vi "Create Gradient Color by Start and End Color DEMO.vi"() -> ()   [LabVIEW 2012, in "Picture Box Tools.lvlib"]
uses:
  Picture Box Tools.lvlib
panel:
  in  "End":u32(colorbox)
  in  "Start":u32(colorbox)=16448250
  out "1 Pix W - Color Box Array":u32[](array[colorbox])=[16448250, 16382457, 16316664, 16250871, 16185078, 16119285, 16053492, 15987699, 15921906, 15856113, 15790320, 15724527, 15658734, 15592941, 15527148, 15461355, 15395562, 15329769, 15263976, 15198183, 15132390, 15066597, 15000804, 14935011, 14869218, 14803425, 14803425, 14737632, 14671839, 14606046, 14540253, 14474460, 14408667, 14342874, 14277081, 14211288, 14145495, 14079702, 14013909, 13948116, 13882323, 13816530, 13750737, 13684944, 13619151, 13553358, 13487565, 13421772, 13355979, 13290186, 13224393, 13158600, 13092807, 13027014, 12961221, 12895428, 12829635, 12763842, 12698049, 12632256, 12566463, 12500670, 12434877, 12369084, 12303291, 12237498, 12171705, 12105912, 12040119, 11974326, 11908533, 11842740, 11776947, 11711154, 11645361, 11579568, 11513775, 11513775, 11447982, 11382189, 11316396, 11250603, 11184810, 11119017, 11053224, 10987431, 10921638, 10855845, 10790052, 10724259, 10658466, 10592673, 10526880, 10461087, 10395294, 10329501, 10263708, 10197915, 10132122, 10066329, 10000536, 9934743, 9868950, 9803157, 9737364, 9671571, 9605778, 9539985, 9474192, 9408399, 9342606, 9276813, 9211020, 9145227, 9079434, 9013641, 8947848, 8882055, 8816262, 8750469, 8684676, 8618883, 8553090, 8487297, 8421504, 8355711, 8289918, 8224125, 8224125, 8158332, 8092539, 8026746, 7960953, 7895160, 7829367, 7763574, 7697781, 7631988, 7566195, 7500402, 7434609, 7368816, 7303023, 7237230, 7171437, 7105644, 7039851, 6974058, 6908265, 6842472, 6776679, 6710886, 6645093, 6579300, 6513507, 6447714, 6381921, 6316128, 6250335, 6184542, 6118749, 6052956, 5987163, 5921370, 5855577, 5789784, 5723991, 5658198, 5592405, 5526612, 5460819, 5395026, 5329233, 5263440, 5197647, 5131854, 5066061, 5000268, 4934475, 4934475, 4868682, 4802889, 4737096, 4671303, 4605510, 4539717, 4473924, 4408131, 4342338, 4276545, 4210752, 4144959, 4079166, 4013373, 3947580, 3881787, 3815994, 3750201, 3684408, 3618615, 3552822, 3487029, 3421236, 3355443, 3289650, 3223857, 3158064, 3092271, 3026478, 2960685, 2894892, 2829099, 2763306, 2697513, 2631720, 2565927, 2500134, 2434341, 2368548, 2302755, 2236962, 2171169, 2105376, 2039583, 1973790, 1907997, 1842204, 1776411, 1710618, 1644825, 1644825, 1579032, 1513239, 1447446, 1381653, 1315860, 1250067, 1184274, 1118481, 1052688, 986895, 921102, 855309, 789516, 723723, 657930, 592137, 526344, 460551, 394758, 328965, 263172, 197379, 131586, 65793, 0]
  out "1 Pix H - Color Box Array":u32[](array[colorbox])=[16448250, 16382457, 16316664, 16250871, 16185078, 16119285, 16053492, 15987699, 15921906, 15856113, 15790320, 15724527, 15658734, 15592941, 15527148, 15461355, 15395562, 15329769, 15263976, 15198183, 15132390, 15066597, 15000804, 14935011, 14869218, 14803425, 14803425, 14737632, 14671839, 14606046, 14540253, 14474460, 14408667, 14342874, 14277081, 14211288, 14145495, 14079702, 14013909, 13948116, 13882323, 13816530, 13750737, 13684944, 13619151, 13553358, 13487565, 13421772, 13355979, 13290186, 13224393, 13158600, 13092807, 13027014, 12961221, 12895428, 12829635, 12763842, 12698049, 12632256, 12566463, 12500670, 12434877, 12369084, 12303291, 12237498, 12171705, 12105912, 12040119, 11974326, 11908533, 11842740, 11776947, 11711154, 11645361, 11579568, 11513775, 11513775, 11447982, 11382189, 11316396, 11250603, 11184810, 11119017, 11053224, 10987431, 10921638, 10855845, 10790052, 10724259, 10658466, 10592673, 10526880, 10461087, 10395294, 10329501, 10263708, 10197915, 10132122, 10066329, 10000536, 9934743, 9868950, 9803157, 9737364, 9671571, 9605778, 9539985, 9474192, 9408399, 9342606, 9276813, 9211020, 9145227, 9079434, 9013641, 8947848, 8882055, 8816262, 8750469, 8684676, 8618883, 8553090, 8487297, 8421504, 8355711, 8289918, 8224125, 8224125, 8158332, 8092539, 8026746, 7960953, 7895160, 7829367, 7763574, 7697781, 7631988, 7566195, 7500402, 7434609, 7368816, 7303023, 7237230, 7171437, 7105644, 7039851, 6974058, 6908265, 6842472, 6776679, 6710886, 6645093, 6579300, 6513507, 6447714, 6381921, 6316128, 6250335, 6184542, 6118749, 6052956, 5987163, 5921370, 5855577, 5789784, 5723991, 5658198, 5592405, 5526612, 5460819, 5395026, 5329233, 5263440, 5197647, 5131854, 5066061, 5000268, 4934475, 4934475, 4868682, 4802889, 4737096, 4671303, 4605510, 4539717, 4473924, 4408131, 4342338, 4276545, 4210752, 4144959, 4079166, 4013373, 3947580, 3881787, 3815994, 3750201, 3684408, 3618615, 3552822, 3487029, 3421236, 3355443, 3289650, 3223857, 3158064, 3092271, 3026478, 2960685, 2894892, 2829099, 2763306, 2697513, 2631720, 2565927, 2500134, 2434341, 2368548, 2302755, 2236962, 2171169, 2105376, 2039583, 1973790, 1907997, 1842204, 1776411, 1710618, 1644825, 1644825, 1579032, 1513239, 1447446, 1381653, 1315860, 1250067, 1184274, 1118481, 1052688, 986895, 921102, 855309, 789516, 723723, 657930, 592137, 526344, 460551, 394758, 328965, 263172, 197379, 131586, 65793, 0]
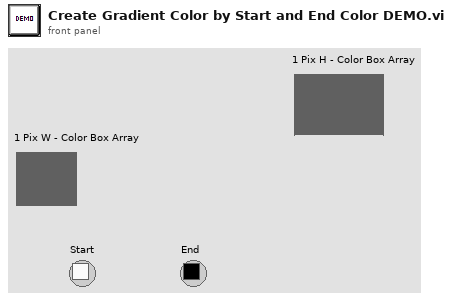
[diagram p1: front panel]
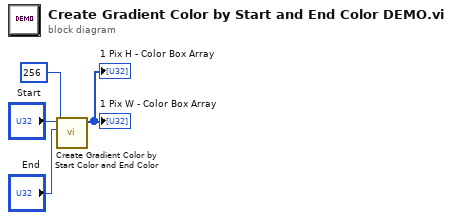
[diagram p0: block diagram]
diagram:
  n1 = call "Create Gradient Color by Start Color and End Color.vi"("Length"=256, "End"="End", "Start"="Start") -> ("ColorArray"=→"1 Pix H - Color Box Array" →"1 Pix W - Color Box Array":u32[])  [unwired: 7 in, 1 out]
